vi "MES.main.xio.vi"() -> ()   [LabVIEW 2014]
uses:
  Ctl.xio/type defs/ini file actions.ctl
  Ctl.xio/type defs/ini entry value.ctl
  Ctl.xio/type defs/ini entry.ctl
  Ctl.xio/type defs/ini entry types.ctl
  <vilib>/Utility/file.llb/Read From Spreadsheet File (string).vi
panel:
  in  "退出系统":bool
  in  "自定义标签":bool
  out "项目名称":string
  in  "用户登录":bool
  in  "Buttons":T1
  in  "分站":T2(tab)
  out "粗切工位生产信息":string[][](table)
  out "热处理工位生产信息":string[][](table)
  out "精切工位生产信息":string[][](table)
  out "PDF焊接工位生产信息":string[][](table)
  out "打凹点\\预载力工位生产信息":string[][](table)
  out "收卷工位生产信息":string[][](table)
  out "EOL检测工位生产信息":string[][](table)
  out "收卷当期项目":string
  out "PDF项目":string
  out "精切项目":string
  out "热处理项目":string
  out "EOL 终检条码（未启用）":string
  out "EOL 当前状态":string
  out "收卷当前状态":string
  out "收卷上料车条码":string
  out "PDF焊接固化料车条码":string
  out "PDF当前状态":string
  out "PDF焊接上料车条码":string
  out "精切当前状态":string
  out "精切下料车条码":string
  out "精切上料车条码":string
  in  "当前项目选择":u16(ring) items=["V254A", "V254B", "C101A", "C101B", "FS11A", "FS11B", "FS11C"]
  out "热处理当前状态":string
  out "热处理出口条码":string
  out "热处理入口条码":string
  out "粗切当前状态":string
  out "粗切条码":string
  out "粗切项目":string
  out "当前时间":string
  out "当前日期":string
  # "汽车遮阳帘生产线"
  # "当前项目"
  # "当前项目"
  # "当前项目"
  # "当前项目"
  # "当前项目"
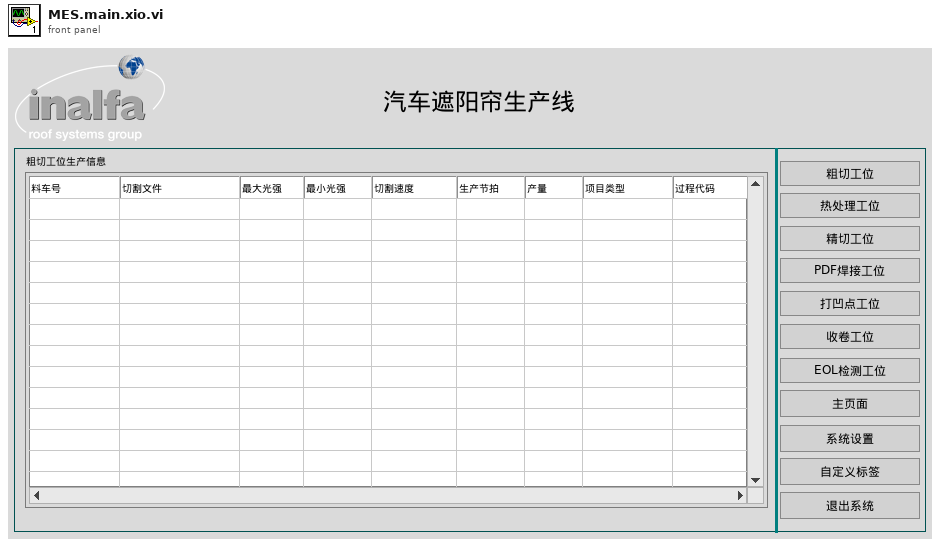
[diagram p1: front panel]
types:
  T1 = cluster{"粗切工位":bool, "热处理工位":bool, "精切工位":bool, "PDF焊接工位":bool, "打凹点工位":bool, "收卷工位":bool, "EOL检测工位":bool, "工位预览":bool}
  T2 = enum32{"粗切工位", "热处理工位", "精切工位", "PDF焊接工位", "打凹点\\预载力工位", "收卷工位", "EOL检测工位", "所有工位预览"}
  T3 = enum32{"产品配置", "粗切工位", "热处理工位", "精切工位", "PDF焊接工位", "打凹点\\预载力工位", "收卷工位", "EOL检测工位", "所有工位预览"}
  T4 = typedef "ini entry.ctl" = cluster{"section":string, "key":string, "type":T5, "default value":T6}
  T5 = typedef "ini entry types.ctl" = enum16{"Boolean", "Double", "I32", "Path", "String", "U32"}
  T6 = typedef "ini entry value.ctl" = cluster{"Boolean":bool, "Dbl":dbl, "I32":i32, "Path":path, "String":string, "U32":u32}
  T7 = typedef "ini file actions.ctl" = enum16{"read ini", "write ini"}
  T8 = cluster{"打凹点\\预载力工位生产信息":refnum<vi>, "项目名称":refnum<vi>}
  T9 = cluster{"粗切工位生产信息":refnum<vi>, "粗切条码":refnum<vi>, "粗切当前状态":refnum<vi>, "粗切项目":refnum<vi>}
  T10 = cluster{"热处理工位生产信息":refnum<vi>, "热处理入口条码":refnum<vi>, "热处理当前状态":refnum<vi>, "热处理出口条码":refnum<vi>, "热处理项目":refnum<vi>}
  T11 = cluster{"精切工位生产信息":refnum<vi>, "精切上料车条码":refnum<vi>, "精切当前状态":refnum<vi>, "精切下料车条码":refnum<vi>, "精切项目":refnum<vi>}
  T12 = cluster{"PDF焊接工位生产信息":refnum<vi>, "PDF焊接上料车条码":refnum<vi>, "PDF当前状态":refnum<vi>, "PDF焊接固化料车条码":refnum<vi>, "PDF项目":refnum<vi>}
  T13 = cluster{"EOL检测工位生产信息":refnum<vi>, "EOL 终检条码（未启用）":refnum<vi>, "EOL 当前状态":refnum<vi>, "项目名称":refnum<vi>}
  T14 = cluster{"收卷工位生产信息":refnum<vi>, "收卷上料车条码":refnum<vi>, "收卷当前状态":refnum<vi>, "收卷当期项目":refnum<vi>}
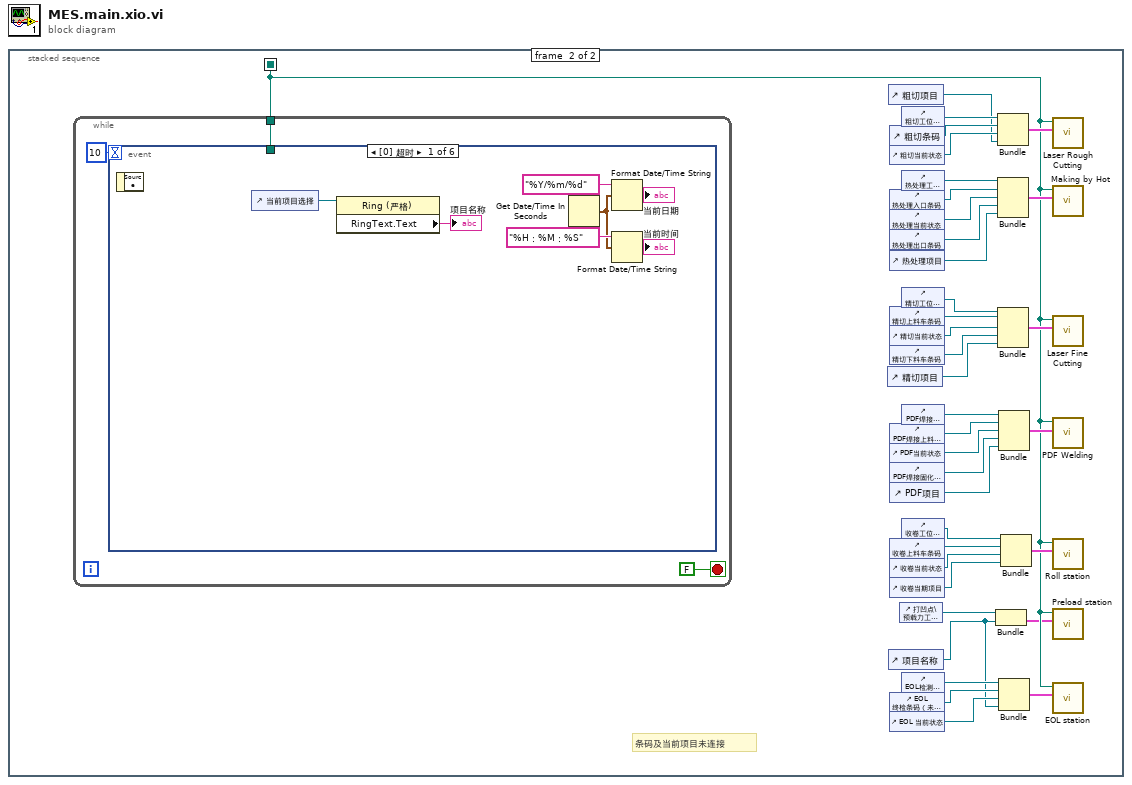
[diagram p0: block diagram]
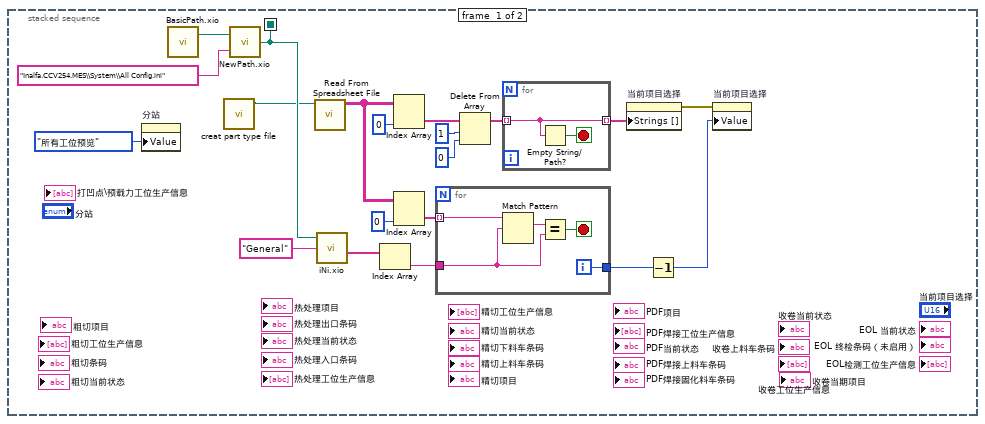
[diagram p2: hidden frame]
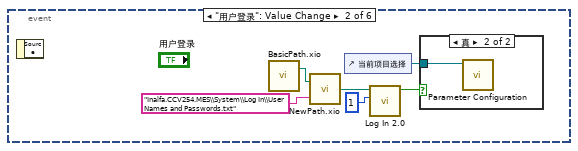
[diagram p3: hidden frame]
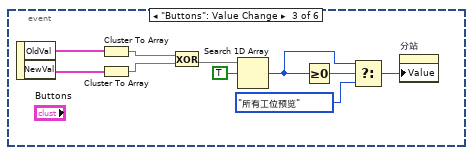
[diagram p5: hidden frame]
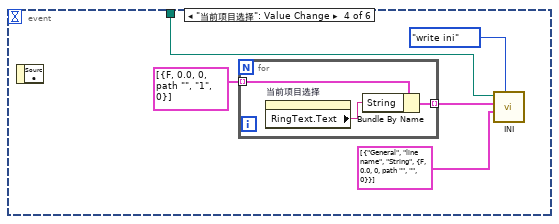
[diagram p6: hidden frame]
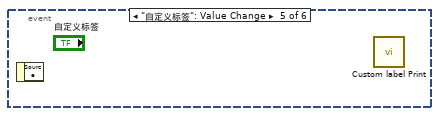
[diagram p7: hidden frame]
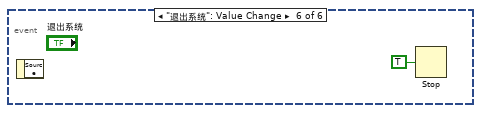
[diagram p8: hidden frame]
diagram:
  n1 = stacked-sequence {
    seq-local: [w12 _] -> [_ w30]
    frame #0 {
      n2 = property on="分站" class="TabCtl (严格)"("Value"=T2."所有工位预览" ("分站")) -> ()  [unwired: 2 in, 2 out]
      n3 = call "BasicPath.xio.vi"() -> ("stripped path"=w19:path)  [unwired: 1 in, 1 out]
      n4 = call "creat part type file.vi"() -> ("new file path (Not A Path if cancelled)"=w1:path)  [unwired: 11 in]
      n5 = call "NewPath.xio.vi"("Append path"="Inalfa.CCV254.MES\\System\\All Config.ini", "Basic path"=w19) -> ("New path"=w12:path)
      n6 = call-poly <vilib>:"Read From Spreadsheet File.vi"("file path (dialog if empty)"=w1) -> ("all rows"=w5:string[][])  [unwired: 6 in, 4 out]
      n7 = call "iNi.xio.vi"("configuration file path"=w12, "Sections"="General") -> ("Values"=w14:string[])  [unwired: 1 in, 4 out]
      n8 = Index Array(array=w14) -> (element=w16:string)  [unwired: 1 in]
      n9 = Index Array(array=w5, index (col)=0 ("禁用的索引 (列)")) -> (element=w8:string[])  [unwired: 1 in]
      n10 = Index Array(array=w5, index (col)=0 ("禁用的索引 (列)")) -> (element=w17:string[])  [unwired: 1 in]
      n11 = for {
        tunnel: w17 -> [w27] mode=indexing
        tunnel: [w24] -> w18
        tunnel: w16 -> [w23]
        i -> [w24]
        stop <- w25 stop-if-true
        n12 = Match Pattern(string=w27, regular expression=w23) -> (match substring=w26:string)  [unwired: 1 in, 3 out]
        n13 = Equal?(x=w26, y=w23) -> (x = y?=w25:bool)
      }
      n14 = Delete From Array(array=w8, length=1 ("长度"), index=0 ("索引")) -> (array with subset deleted=w6:string[])  [unwired: 1 out]
      n15 = for {
        tunnel: w6 -> [w21] mode=indexing
        tunnel: [w21] -> w2 mode=indexing
        stop <- w22 stop-if-true
        n16 = Empty String/Path?(string/path=w21) -> (empty?=w22:bool)
      }
      n17 = property on="当前项目选择" class="Ring (严格)"("Strings []"=w2) -> (error out=w4:errorcluster)  [unwired: 2 in, 1 out]
      n18 = Decrement(x=w18) -> (x-1=w3:i32)
      n19 = property on="当前项目选择" class="Ring (严格)"(error in=w4, "Value"=w3) -> ()  [unwired: 1 in, 2 out]
    }
    frame #1 {
      # "条码及当前项目未连接"
      n20 = while {
        tunnel: w30 -> [w64]
        stop <- FALSE stop-if-true
        n21 = event shown="[0] 超时" {
          selector: _ -> [_ _ _ _ _ _]
          dyn-events: _ -> [_ _ _ _ _ _]
          timeout: 10 -> [_ _ _ _ _ _]
          tunnel: w64 -> [_ _ _ w91 _ _]
          event Timeout {
            n22 = event-data() -> ()  [unwired: 1 in, 1 out]
            n23 = control-ref of="当前项目选择"() -> (w68:refnum<vi>)
            n24 = property class="Ring (严格)"(reference=w68) -> ("RingText.Text"=→"项目名称":string)  [unwired: 1 in, 2 out]
            n25 = Get Date/Time In Seconds() -> (seconds since 1Jan1904=w72:timestamp)
            n26 = Format Date/Time String(time format string (%c)="%Y/%m/%d" ("时间格式字符串(%c)"), seconds (now)=w72) -> (date/time string=→"当前日期":string)  [unwired: 1 in]
            n27 = Format Date/Time String(time format string (%c)="%H：%M：%S" ("时间格式字符串(%c)"), seconds (now)=w72) -> (date/time string=→"当前时间":string)  [unwired: 1 in]
          }
          event "用户登录": Value Change {
            n28 = event-data() -> ()  [unwired: 1 in, 1 out]
            n29 = call "BasicPath.xio.vi"() -> ("stripped path"=w78:path)  [unwired: 1 in, 1 out]
            n30 = call "NewPath.xio.vi"("Append path"="Inalfa.CCV254.MES\\System\\Log In\\User Names and Passwords.txt", "Basic path"=w78) -> ("New path"=w77:path)
            n31 = control-ref of="当前项目选择"() -> (w74:refnum<vi>)
            n32 = call "Log In 2.0.vi"("required access level"=1, "Program Root Path"=w77) -> ("passed"=w75:bool)  [unwired: 6 in, 3 out]
            n33 = case shown="真" w75 {
              tunnel: w74 -> [_ w80]
              frame False {
              }
              frame True {
                n34 = call "Parameter Configuration.vi"("当前项目选择"=w80) -> ()  [unwired: 11 in]
              }
            }
          }
          event "Buttons": Value Change {
            n35 = event-data() -> ("OldVal"=w90:T1, "NewVal"=w89:T1)  [unwired: 1 in]
            n36 = Cluster To Array(cluster=w90) -> (array=w88:bool[])
            n37 = Cluster To Array(cluster=w89) -> (array=w87:bool[])
            n38 = Exclusive Or(1:w87, 2:w88) -> (0:w86:bool[])
            n39 = Search 1D Array(1D array=w86, element=TRUE) -> (index of element=w81:i32)  [unwired: 1 in]
            n40 = Greater Or Equal To 0?(x=w81) -> (x >= 0?=w84:bool)
            n41 = Select(t=w81, s=w84, f=T3."所有工位预览" ("分站")) -> (s? t:f=w83:u32)
            n42 = property on="分站" class="TabCtl (严格)"("Value"=w83) -> ()  [unwired: 2 in, 2 out]
          }
          event "当前项目选择": Value Change {
            n43 = event-data() -> ()  [unwired: 1 in, 1 out]
            n44 = for {
              tunnel: T6[] [{"Boolean"=FALSE, "Dbl"=0.0, "I32"=0, "Path"=path "", "String"="1", "U32"=0}] ("values in") -> [w98] mode=indexing
              tunnel: [w96] -> w92 mode=indexing
              n45 = property on="当前项目选择" class="Ring (严格)"() -> ("RingText.Text"=w97:string)  [unwired: 2 in, 2 out]
              n46 = Bundle By Name(cluster=w98, "String"=w97) -> (w96:T6)
            }
            n47 = call "INI.vi"("configuration file path"=w91, "action"=ini_file_actions."write ini", "values in"=w92, "ini entry descriptors"=T4[] [{"section"="General", "key"="line name", "type"=enum."String", "default value"={"Boolean"=FALSE, "Dbl"=0.0, "I32"=0, "Path"=path "", "String"="", "U32"=0}}]) -> ()  [unwired: 2 in, 3 out]
          }
          event "自定义标签": Value Change {
            n48 = event-data() -> ()  [unwired: 1 in, 1 out]
            n49 = call "Custom label Print.vi"() -> ()  [unwired: 12 in]
          }
          event "退出系统": Value Change {
            n50 = event-data() -> ()  [unwired: 1 in, 1 out]
            n51 = Stop(stop? (T)=TRUE ("停止？(T)")) -> ()
          }
        }
      }
      n52 = control-ref of="精切项目"() -> (w36:refnum<vi>)
      n53 = control-ref of="粗切项目"() -> (w32:refnum<vi>)
      n54 = control-ref of="项目名称"() -> (w28:refnum<vi>)
      n55 = control-ref of="粗切条码"() -> (w62:refnum<vi>)
      n56 = control-ref of="粗切当前状态"() -> (w61:refnum<vi>)
      n57 = control-ref of="热处理入口条码"() -> (w60:refnum<vi>)
      n58 = control-ref of="热处理当前状态"() -> (w58:refnum<vi>)
      n59 = control-ref of="热处理出口条码"() -> (w57:refnum<vi>)
      n60 = control-ref of="热处理项目"() -> (w35:refnum<vi>)
      n61 = control-ref of="精切上料车条码"() -> (w54:refnum<vi>)
      n62 = control-ref of="精切当前状态"() -> (w53:refnum<vi>)
      n63 = control-ref of="精切下料车条码"() -> (w52:refnum<vi>)
      n64 = control-ref of="PDF焊接上料车条码"() -> (w48:refnum<vi>)
      n65 = control-ref of="PDF当前状态"() -> (w47:refnum<vi>)
      n66 = control-ref of="PDF焊接固化料车条码"() -> (w45:refnum<vi>)
      n67 = control-ref of="PDF项目"() -> (w34:refnum<vi>)
      n68 = control-ref of="收卷上料车条码"() -> (w42:refnum<vi>)
      n69 = control-ref of="收卷当前状态"() -> (w41:refnum<vi>)
      n70 = control-ref of="收卷当期项目"() -> (w33:refnum<vi>)
      n71 = control-ref of="EOL 终检条码（未启用）"() -> (w37:refnum<vi>)
      n72 = control-ref of="EOL 当前状态"() -> (w38:refnum<vi>)
      n73 = control-ref of="打凹点\\预载力工位生产信息"() -> (w31:refnum<vi>)
      n74 = control-ref of="粗切工位生产信息"() -> (w63:refnum<vi>)
      n75 = control-ref of="热处理工位生产信息"() -> (w59:refnum<vi>)
      n76 = control-ref of="精切工位生产信息"() -> (w50:refnum<vi>)
      n77 = control-ref of="PDF焊接工位生产信息"() -> (w49:refnum<vi>)
      n78 = control-ref of="收卷工位生产信息"() -> (w43:refnum<vi>)
      n79 = control-ref of="EOL检测工位生产信息"() -> (w39:refnum<vi>)
      n80 = Bundle("打凹点\\预载力工位生产信息"=w31, "项目名称"=w28) -> (w29:T8)  [unwired: 1 in]
      n81 = Bundle("粗切工位生产信息"=w63, "粗切条码"=w62, "粗切当前状态"=w61, "粗切项目"=w32) -> (w56:T9)  [unwired: 1 in]
      n82 = Bundle("热处理工位生产信息"=w59, "热处理入口条码"=w60, "热处理当前状态"=w58, "热处理出口条码"=w57, "热处理项目"=w35) -> (w55:T10)  [unwired: 1 in]
      n83 = Bundle("精切工位生产信息"=w50, "精切上料车条码"=w54, "精切当前状态"=w53, "精切下料车条码"=w52, "精切项目"=w36) -> (w51:T11)  [unwired: 1 in]
      n84 = Bundle("PDF焊接工位生产信息"=w49, "PDF焊接上料车条码"=w48, "PDF当前状态"=w47, "PDF焊接固化料车条码"=w45, "PDF项目"=w34) -> (w46:T12)  [unwired: 1 in]
      n85 = Bundle("EOL检测工位生产信息"=w39, "EOL 终检条码（未启用）"=w37, "EOL 当前状态"=w38, "项目名称"=w28) -> (w40:T13)  [unwired: 1 in]
      n86 = Bundle("收卷工位生产信息"=w43, "收卷上料车条码"=w42, "收卷当前状态"=w41, "收卷当期项目"=w33) -> (w44:T14)  [unwired: 1 in]
      n87 = call "Laser Rough Cutting.vi"("configuration file path"=w30, "rough cutting msic"=w56) -> ()  [unwired: 4 in]
      n88 = call "Making by Hot.vi"("configuration file path"=w30, "making by hot msic inf"=w55) -> ()  [unwired: 4 in]
      n89 = call "Laser Fine Cutting.vi"("configuration file path"=w30, "fine cutting msic"=w51) -> ()  [unwired: 4 in]
      n90 = call "PDF Welding.vi"("configuration file path"=w30, "PDF Welding msic inf"=w46) -> ()  [unwired: 4 in]
      n91 = call "Roll station.vi"("configuration file path"=w30, "Roll station msic inf"=w44) -> ()  [unwired: 4 in]
      n92 = call "Preload station.vi"("configuration file path"=w30, "Preload station msic inf"=w29) -> ()  [unwired: 4 in]
      n93 = call "EOL station.vi"("configuration file path"=w30, "EOL station msic inf"=w40) -> ()  [unwired: 4 in]
    }
  }
